vi "Set Analog Replay Data Options.vi"(8 "error in (no error)":errorcluster, 10 "Analog Replay Data Options":T1={"Selected File"=path "", "Group"="", "Channel"="", "DataPlugin"="", "ReverseData"=FALSE, "DispTwoRotations"=FALSE, "FPGA memory size"=enum."16,384", "CycleAngle?"=enum."Crank angle", "Data Selection Method"=enum."Manual", "File start offset"=1, "Samples"=1, "Missing teeth location (degrees)"=1.0} {"Missing teeth location (degrees)" min=0.0; "Samples" min=1; "File start offset" min=0}, 11 "NodeID":u64) -> (0 "error out":errorcluster, 3 "NodeID":u64)   [LabVIEW 2015, in "Engine Simulation Toolkit Scripting API.lvlib"]
uses:
  Engine Simulation Toolkit Scripting API.lvlib
  Analog Replay Data Options.ctl
  System Explorer/FPGA Mem Size.ctl
  System Explorer/Position Reference.ctl
  System Explorer/Data Replay Data Selection Method.ctl
  System Explorer/File Load Dialog.ctl
  <vilib>/Platform/storage/utility/usiPluginInformation.ctl
  System Explorer/Engine Simulation Toolkit System Explorer.lvlib
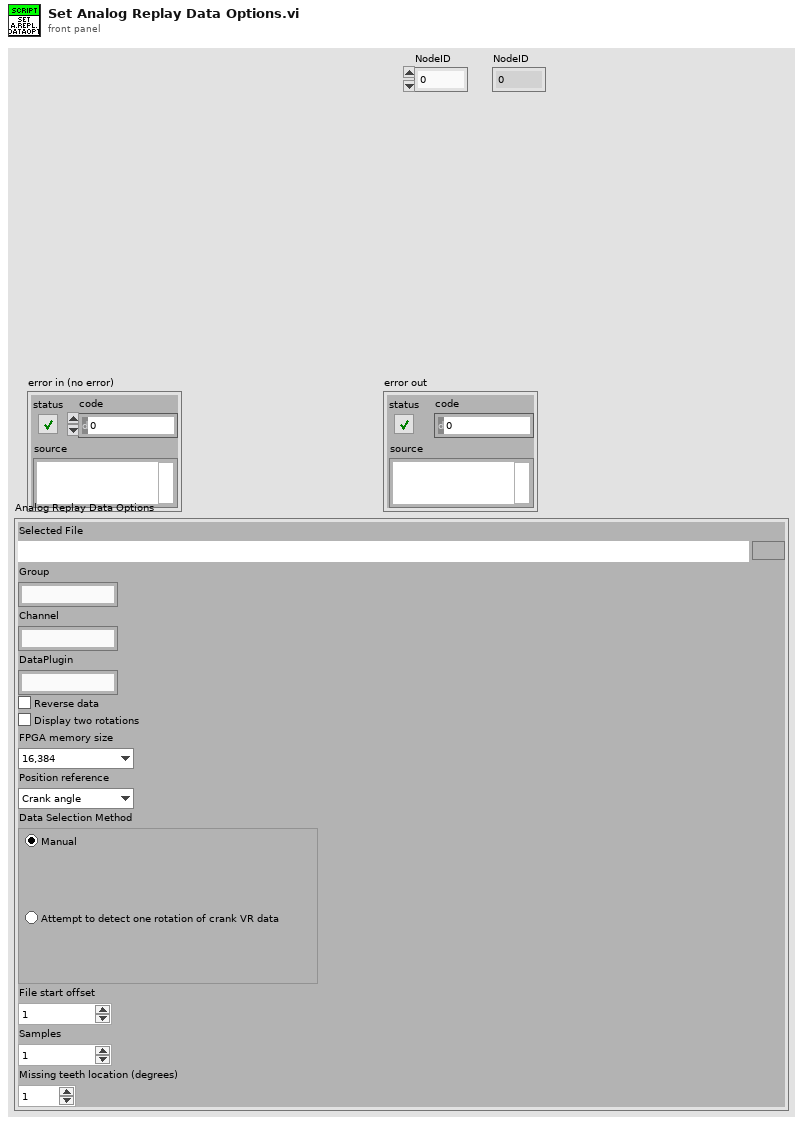
[diagram p1: front panel]
types:
  T1 = typedef "Engine Simulation Toolkit Scripting API.lvlib/Analog Replay Data Options.ctl" = cluster{"Selected File":path, "Group":string, "Channel":string, "DataPlugin":string, "ReverseData":bool, "DispTwoRotations":bool, "FPGA memory size":T2, "CycleAngle?":T3, "Data Selection Method":T4, "File start offset":i32, "Samples":i32, "Missing teeth location (degrees)":dbl}
  T2 = typedef "Engine Simulation Toolkit System Explorer.lvlib/FPGA Mem Size.ctl" = enum16{"65,536", "32,768", "16,384", "8,192", "4,096", "2,048", "1,024"}
  T3 = typedef "Engine Simulation Toolkit System Explorer.lvlib/Position Reference.ctl" = enum16{"Crank angle", "Cycle angle"}
  T4 = typedef "Engine Simulation Toolkit System Explorer.lvlib/Data Replay Data Selection Method.ctl" = enum32{"Manual", "AutoVRCrank"}
  T5 = typedef "Engine Simulation Toolkit System Explorer.lvlib/File Load Dialog.ctl" = cluster{"File":path, "Group":string, "Channel":string, "DataPlugin":string, "MissingTeeth":dbl, "ErrState":string, "File Selected":bool, "Data Selection Method":T4, "Offset":i32, "Length":i32, "DataPlugins Info":T6[], "Controls":refnum<vi>[], "File Ref":refnum<k20>, "Groups":string[], "Channels":string[], "Groups Refs":refnum<k20>[], "Channel Refs":refnum<k20>[], "Cancelled":bool, "Position reference":T3, "FPGA memory size":T2, "GroupRef":refnum<k20>, "ChanRef":refnum<k20>, "Data":dbl[], "ReverseData":bool, "DispTwoRotations":bool, "cycle range":u16}
  T6 = typedef "usiPluginInformation.ctl" = cluster{"name":string, "version":string, "type":string, "read-only?":bool, "extensions":string[]}
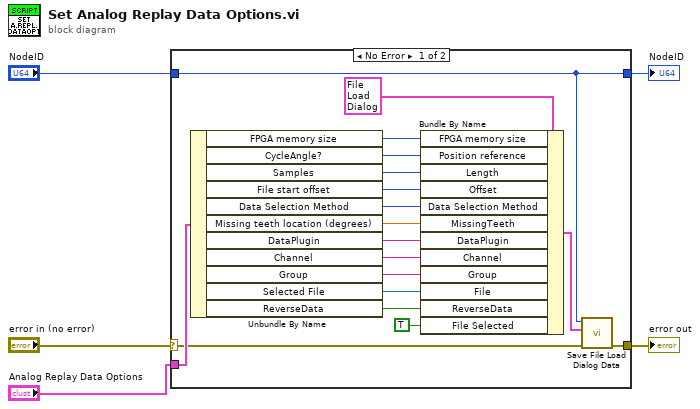
[diagram p0: block diagram]
diagram:
  n1 = case shown="No Error" "error in (no error)" {
    selector: "error in (no error)" -> [w8 w25]
    tunnel: "Analog Replay Data Options" -> [w23 _]
    tunnel: "NodeID" -> [w6 w24]
    tunnel: [w7 w25] -> w2
    tunnel: [w6 w24] -> w1
    frame No Error {
      n2 = Unbundle By Name(w23) -> ("FPGA memory size"=w22:T2, "CycleAngle?"=w21:T3, "Samples"=w19:i32, "File start offset"=w20:i32, "Data Selection Method"=w18:T4, "Missing teeth location (degrees)"=w17:dbl, "DataPlugin"=w12:string, "Channel"=w13:string, "Group"=w14:string, "Selected File"=w15:path, "ReverseData"=w16:bool)
      n3 = Bundle By Name(cluster=T5 {"File"=path "", "Group"="", "Channel"="", "DataPlugin"="", "MissingTeeth"=0.0, "ErrState"="", "File Selected"=FALSE, "Data Selection Method"=enum."Manual", "Offset"=0, "Length"=0, "DataPlugins Info"=[], "Controls"=[], "File Ref"=refnum, "Groups"=[], "Channels"=[], "Groups Refs"=[], "Channel Refs"=[], "Cancelled"=FALSE, "Position reference"=enum."Crank angle", "FPGA memory size"=enum."32,768", "GroupRef"=refnum, "ChanRef"=refnum, "Data"=[], "ReverseData"=FALSE, "DispTwoRotations"=FALSE, "cycle range"=720} ("FileDialog"), "FPGA memory size"=w22, "Position reference"=w21, "Length"=w19, "Offset"=w20, "Data Selection Method"=w18, "MissingTeeth"=w17, "DataPlugin"=w12, "Channel"=w13, "Group"=w14, "File"=w15, "ReverseData"=w16, "File Selected"=TRUE) -> (w9:T5)
      n4 = call "Save File Load Dialog Data.vi"("error in (no error)"=w8, "FileDialog"=w9, "Node Ptr"=w6) -> ("error out"=w7:errorcluster)  [unwired: 8 in]
    }
    frame Error {
    }
  }
  "error out" <- w2
  "NodeID" <- w1
